vi "p21_b.vi"(2 "fs muestreo":dbl, 3 "tsim":dbl) -> (0 "T":dbl, 1 "NS":dbl)   [LabVIEW 2023]
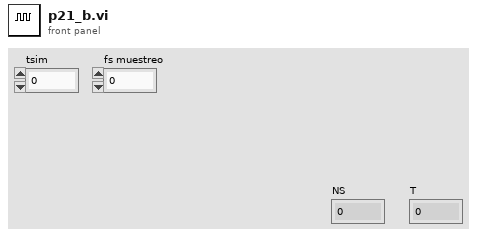
[diagram p1: front panel]
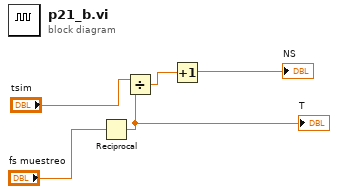
[diagram p0: block diagram]
diagram:
  n1 = Reciprocal(x="fs muestreo") -> (1/x=w3:dbl)
  "T" <- w3
  n2 = Divide(x="tsim", y=w3) -> (x/y=w4:dbl)
  n3 = Increment(x=w4) -> (x+1=→"NS":dbl)
